vi "Convert Measured Rate.vi"(2 "FPGA Clock Rate (Hz)":dbl, 3 "Measured Reference Time Period (Ticks)":u32) -> (0 "Measured Reference Loop Rate (kHz)":dbl, 1 "Measured Reference Loop Period (s)":dbl)   [LabVIEW 2015]
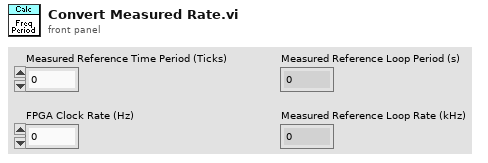
[diagram p1: front panel]
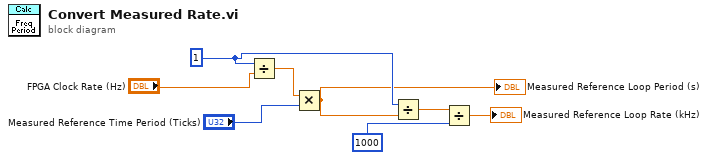
[diagram p0: block diagram]
diagram:
  w7 = 1
  n1 = Divide(x=w7, y="FPGA Clock Rate (Hz)") -> (x/y=w6:dbl)
  n2 = Multiply(x=w6, y="Measured Reference Time Period (Ticks)") -> (x*y=w2:dbl)
  "Measured Reference Loop Period (s)" <- w2
  n3 = Divide(x=w7, y=w2) -> (x/y=w3:dbl)
  n4 = Divide(x=w3, y=1000) -> (x/y=→"Measured Reference Loop Rate (kHz)":dbl)
